vi "Get-lasing.vi"(8 "error in (no error)":errorcluster, 11 "Object ref in":T1) -> (0 "error out":errorcluster, 2 "Lasing?":bool, 3 "Object ref out":T1)   [LabVIEW 2013, in "SLMControl.lvlib" / "SC-Main.lvclass"]
uses:
  SC-Main.lvclass
  Object-reference.ctl
  SC-Main.lvclass/SC-Main.ctl
  Read Lasing notif.vi
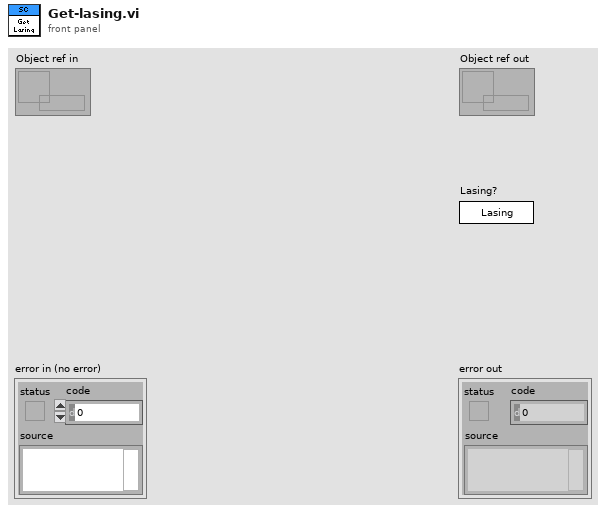
[diagram p1: front panel]
types:
  T1 = typedef "SLMControl.lvlib/SC-Main.lvclass/Object-reference.ctl" = refnum<data-value>
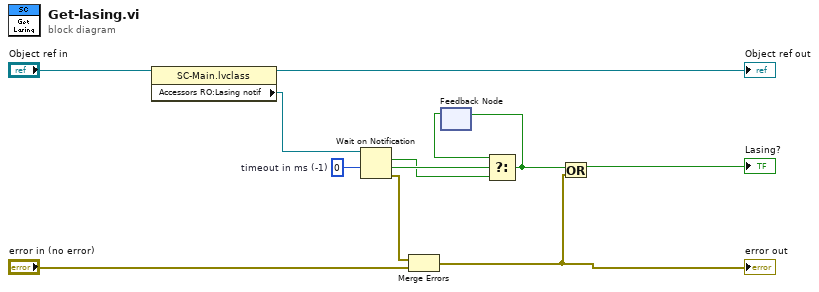
[diagram p0: block diagram]
diagram:
  w7 = 0  # timeout in ms (-1)
  n1 = property class="SC-Main.lvclass"(reference="Object ref in") -> (reference out=→"Object ref out":T1, "Accessors RO:Lasing notif"=w8:refnum<notifier>)  [unwired: 1 in, 1 out]
  n2 = Wait on Notification(notifier=w8, timeout in ms (-1)=w7) -> (notification=w5:bool, timed out?=w6:bool, error out=w12:errorcluster)  [unwired: 2 in, 1 out]
  n3 = Merge Errors(w12, "error in (no error)") -> (w1:errorcluster)
  "error out" <- w1
  n4 = feedback #1() -> (w4:bool)  [unwired: 1 in]
  n5 = Select(t=w4, s=w6, f=w5) -> (s? t:f=w9:bool)
  n6 = feedback-in #1(w9) -> ()
  n7 = Or(x=w9, y=w1) -> (x .or. y?=→"Lasing?":bool)
